vi "source Read.vi"(4 "error in (no error)":errorcluster, 6 "Container State":T6, 7 "Display State In":T4={"Z_Source"={"connect"=FALSE, "Z_Source"=enum."initialize", "Z_State_heating"=enum."on"}, "Write"=FALSE, "Z1_ind"=0, "button state"=enum."init", "reset_timer"=FALSE, "load_timer"=FALSE, "end_timer"=TRUE}) -> (0 "error out":errorcluster, 2 "Value":T3={"connect"=FALSE, "Z_Source"=enum."initialize", "Z_State_heating"=enum."on"}, 3 "Display State Out":T4={"Z_Source"={"connect"=FALSE, "Z_Source"=enum."initialize", "Z_State_heating"=enum."on"}, "Write"=FALSE, "Z1_ind"=0, "button state"=enum."init", "reset_timer"=FALSE, "load_timer"=FALSE, "end_timer"=TRUE})   [LabVIEW 2019, in "Heating.lvlib" / "Z_OnSwitch.xctl"]
uses:
  Z_OnSwitch.xctl
  <vilib>/_xctls/Container State.ctl
  State.ctl
  Y_source.ctl
  Z_State.ctl
  On_ButtonState.ctl
  <vilib>/_xctls/XControlSupport.lvlib
  Heating.lvlib
panel:
  # "Replace the Value Indicator below with an Indicator of desired type.\nDo not remove this Indicator or the others from the connector pane. \nDo not change the connector pane pattern.\nThe Value Indicator should always be the second terminal from top on the output side in the connector pane."
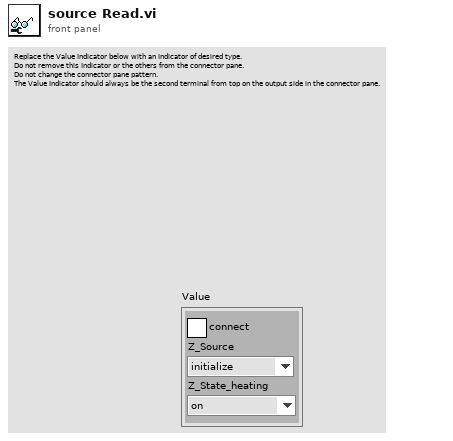
[diagram p1: front panel]
types:
  T1 = typedef "Heating.lvlib/Y_source.ctl" = enum8{"initialize", "local disabled", "local hand", "hand", "auto", "dist"}
  T2 = typedef "Heating.lvlib/Z_State.ctl" = enum8{"initialization", "alarm", "disabled", "not ready", "stop ready", "reserv", "switched off", "reserv2", "switched on", "check", "on min", "decrease out", "on", "increase out", "on max"}
  T3 = cluster{"connect":bool, "Z_Source":T1, "Z_State_heating":T2}
  T4 = typedef "Heating.lvlib/Z_OnSwitch.xctl/State.ctl" = cluster{"Z_Source":cluster{"connect":bool, "Z_Source":T1, "Z_State_heating":T2}, "Write":bool, "Z1_ind":u8, "button state":T5, "reset_timer":bool, "load_timer":bool, "end_timer":bool}
  T5 = typedef "Heating.lvlib/Z_OnSwitch.xctl/On_ButtonState.ctl" = enum16{"init", "not connect", "local disabled", "local hand", "switch off", "off", "switch on", "on", "auto", "dist"}
  T6 = typedef "XControlSupport.lvlib/Container State.ctl" = cluster{"Indicator?":bool, "Run Mode?":bool, " Refnum":refnum<vi>}
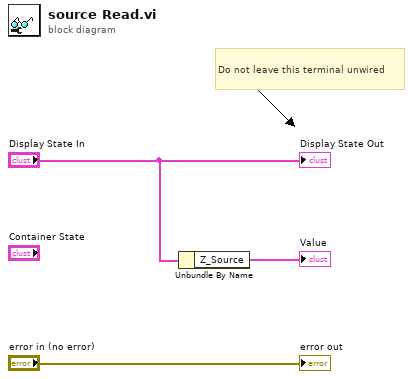
[diagram p0: block diagram]
diagram:
  # "Do not leave this terminal unwired"
  n1 = Unbundle By Name("Display State In") -> ("Z_Source"=→"Value":T3)
  "error out" <- "error in (no error)"
  "Display State Out" <- "Display State In"
